vi "Utilities_Remove_TDMS_Files.vi"() -> ()   [LabVIEW 2020]
panel:
  out "data":string[](array[string])
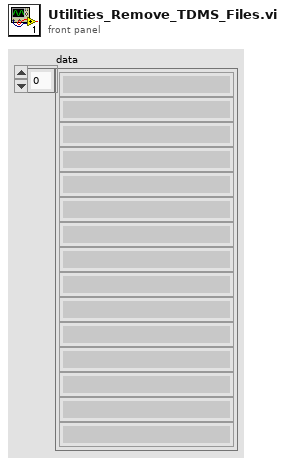
[diagram p1: front panel]
types:
  T1 = enum16{"open", "open or create", "create or replace", "create", "open (read-only)"}
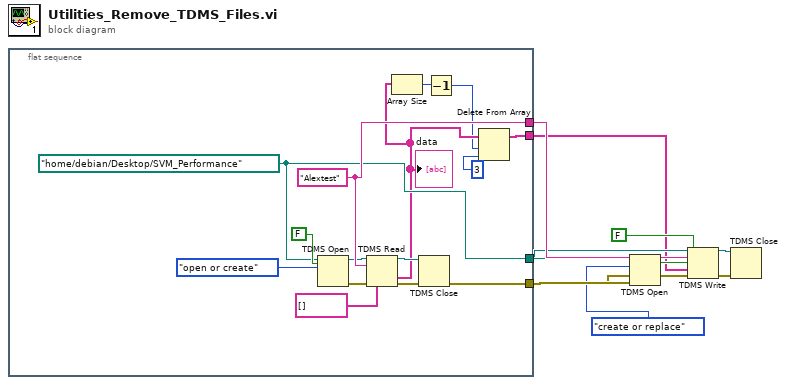
[diagram p0: block diagram]
diagram:
  n1 = flat-sequence {
    tunnel: [w21] -> w8
    tunnel: [w19] -> w1
    tunnel: [w16] -> w7
    tunnel: [w15] -> w6
    frame #0 {
      w15 = path "/home/debian/Desktop/SVM_Performance" ("base path")
      w21 = "Alextest" ("group name in (Untitled)")
      n2 = TDMS Open(5:FALSE ("create index file? (T)"), 10:T1."open or create" ("operation (0:open)"), 11:w15) -> (0:w23:errorcluster, 3:w20:refnum<k34>)  [unwired: 4 in]
      n3 = TDMS Read(0:w20, 5:w21, 11:w23, 12:string[] []) -> (4:w17:refnum<k34>, 10:w13:string[], 15:w18:errorcluster)  [unwired: 4 in, 3 out]
      "data" <- w13
      n4 = Array Size(array=w13) -> (size(s)=w12:i32)
      n5 = TDMS Close(8:w18, 11:w17) -> (0:w16:errorcluster)  [unwired: 1 out]
      n6 = Decrement(x=w12) -> (x-1=w11:i32)
      n7 = Delete From Array(array=w13, length=w11, index=3) -> (array with subset deleted=w19:string[])  [unwired: 1 out]
    }
  }
  n8 = TDMS Open(5:FALSE ("create index file? (T)"), 8:w7, 10:T1."create or replace" ("operation (0:open)"), 11:w6) -> (0:w4:errorcluster, 3:w3:refnum<k34>)  [unwired: 3 in]
  n9 = TDMS Write(0:w3, 5:w8, 9:w1, 11:w4) -> (4:w9:refnum<k34>, 15:w10:errorcluster)  [unwired: 2 in, 2 out]
  n10 = TDMS Close(8:w10, 11:w9) -> ()  [unwired: 2 out]
